vi "Config Seq & Error.vi"(8 "error in (no error)":errorcluster, 11 "Sequences":T1) -> (0 "error out":errorcluster, 3 "Sequences":T1)   [LabVIEW 2014, in "SeqLoop.lvlib"]
uses:
  TypeDefs/Sequence.ctl
  TypeDefs/STEP.ctl
  TypeDefs/LogicParsedExpression.ctl
  Mimico Display/TypeDefs/Mimic Data.ctl
  Mimico Display/TypeDefs/BG Image.ctl
  Mimico Display/TypeDefs/mObject.ctl
  SeqLoop.lvlib
  Mimico Display/Mimico Display.lvlib
panel:
  in  "Save":bool
  in  "Close":bool
  in  "Config AutoZero":bool
  in  "Error&Alarms":bool
  # "Elija la opción que desea configurar"
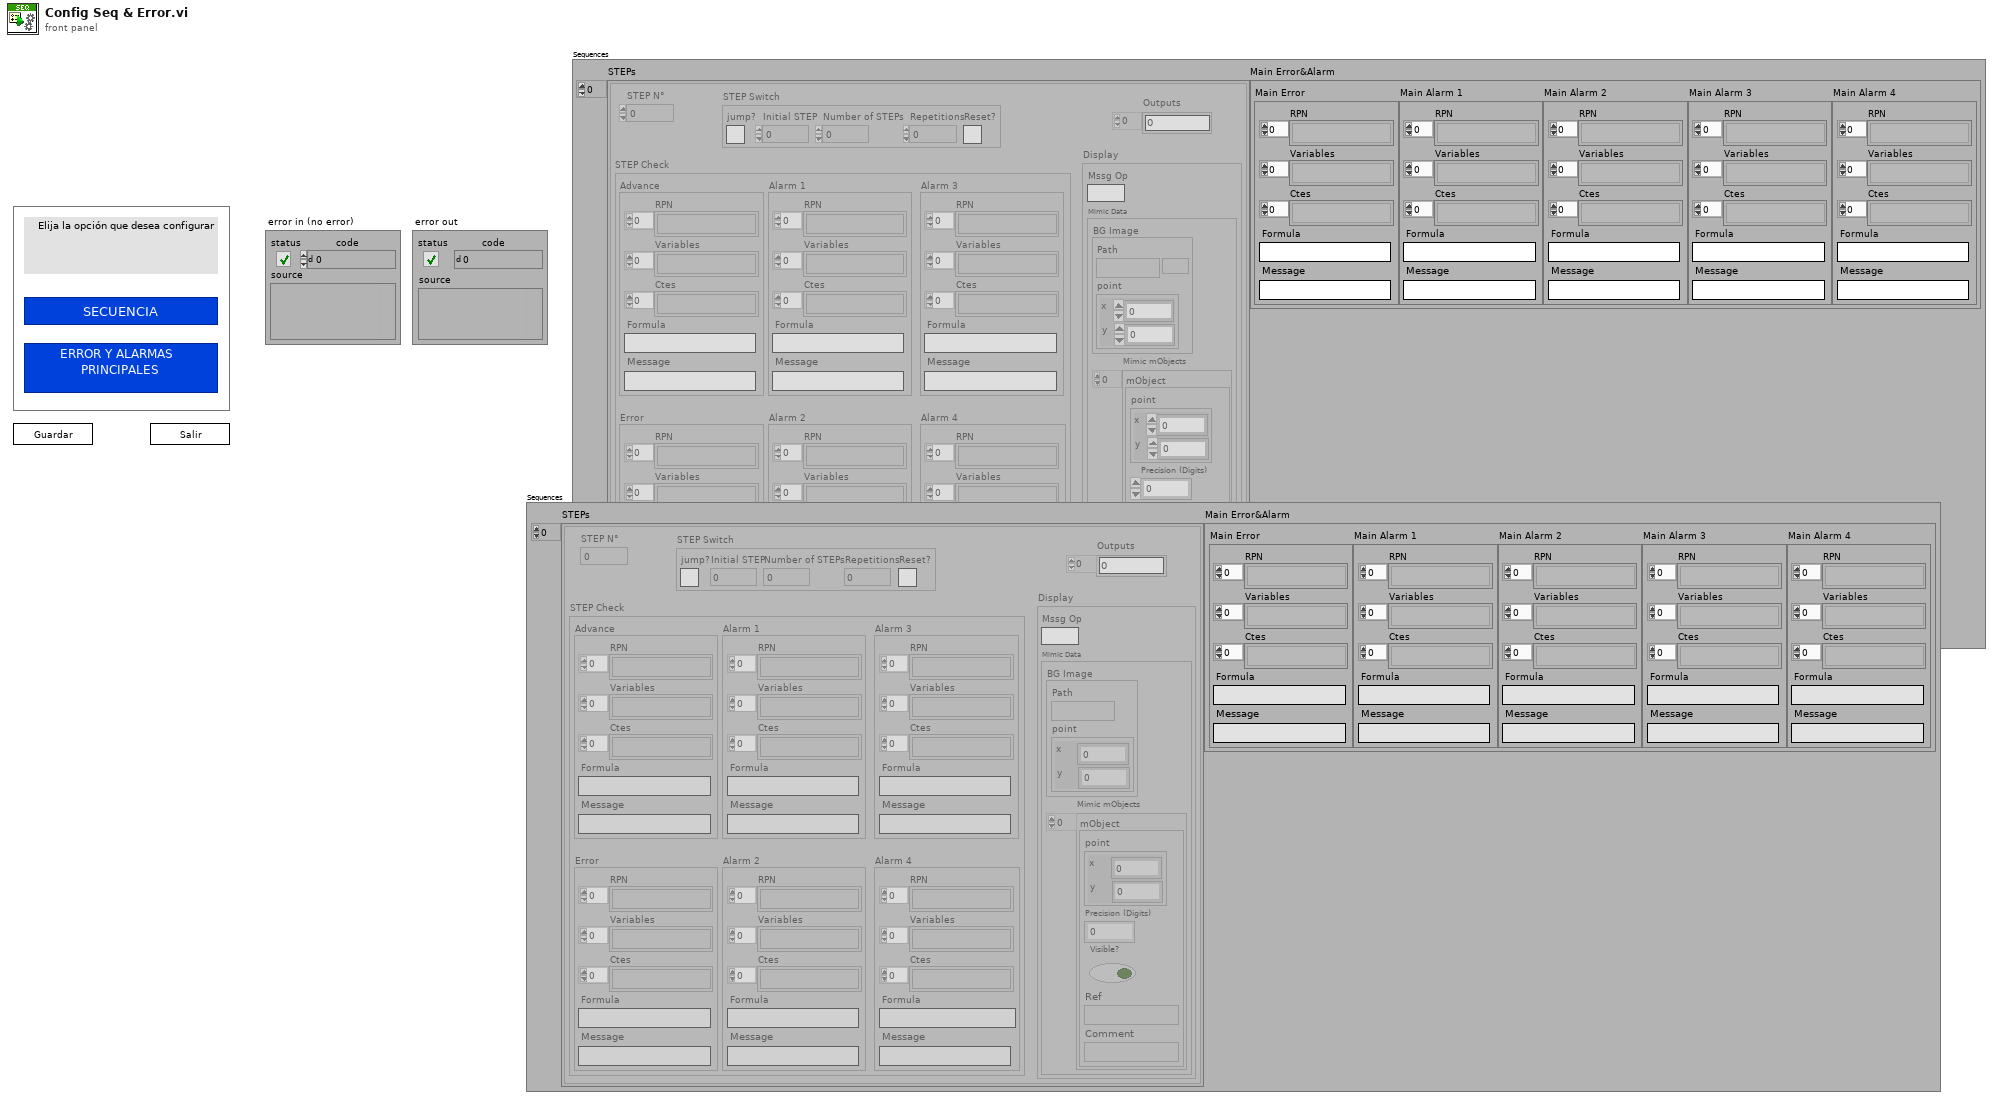
[diagram p1: front panel]
types:
  T1 = typedef "SeqLoop.lvlib/Sequence.ctl" = cluster{"STEPs":T2[], "Main Error&Alarm":cluster{"Main Error":T3, "Main Alarm 1":T3, "Main Alarm 2":T3, "Main Alarm 3":T3, "Main Alarm 4":T3}}
  T2 = typedef "SeqLoop.lvlib/STEP.ctl" = cluster{"STEP N°":u32, "STEP Switch":cluster{"jump?":bool, "Initial STEP":u32, "Number of STEPs":u32, "Repetitions":u32, "Reset?":bool}, "Outputs":i32[], "STEP Check":cluster{"Advance":T3, "Error ":T3, "Alarm 1":T3, "Alarm 2":T3, "Alarm 3":T3, "Alarm 4":T3}, "Display":cluster{"Mssg Op":string, "Mimic Data":T4}}
  T3 = typedef "SeqLoop.lvlib/LogicParsedExpression.ctl" = cluster{"RPN ":string[], "Variables":string[], "Ctes":string[], "Formula":string, "Message":string}
  T4 = typedef "SeqLoop.lvlib/Mimico Display.lvlib/Mimic Data.ctl" = cluster{"BG Image":T5, "Mimic mObjects":T6[]}
  T5 = typedef "SeqLoop.lvlib/Mimico Display.lvlib/BG Image.ctl" = cluster{"Path":path, "point":cluster{"x":i16, "y":i16}}
  T6 = typedef "SeqLoop.lvlib/Mimico Display.lvlib/mObject.ctl" = cluster{"point":cluster{"x":i16, "y":i16}, "Precision (Digits)":i32, "Visible?":bool, "Ref":string, "Comment":string}
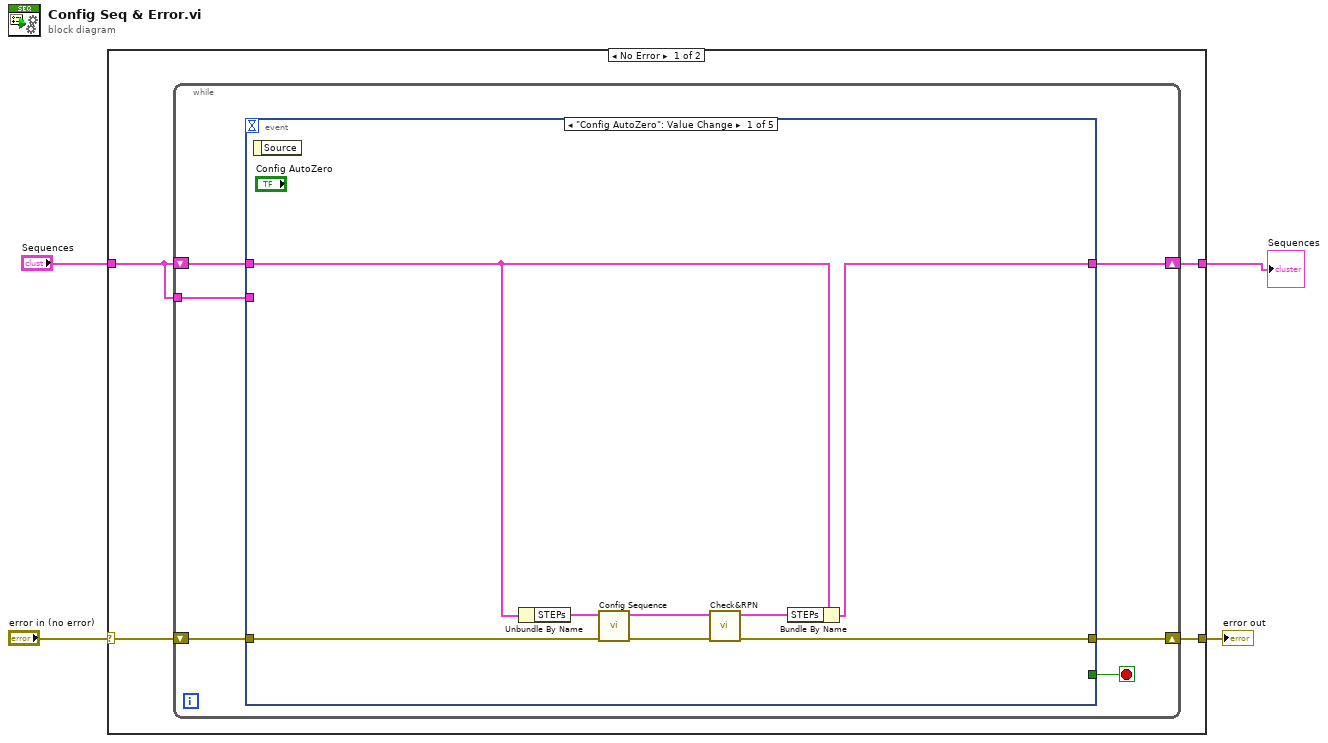
[diagram p0: block diagram]
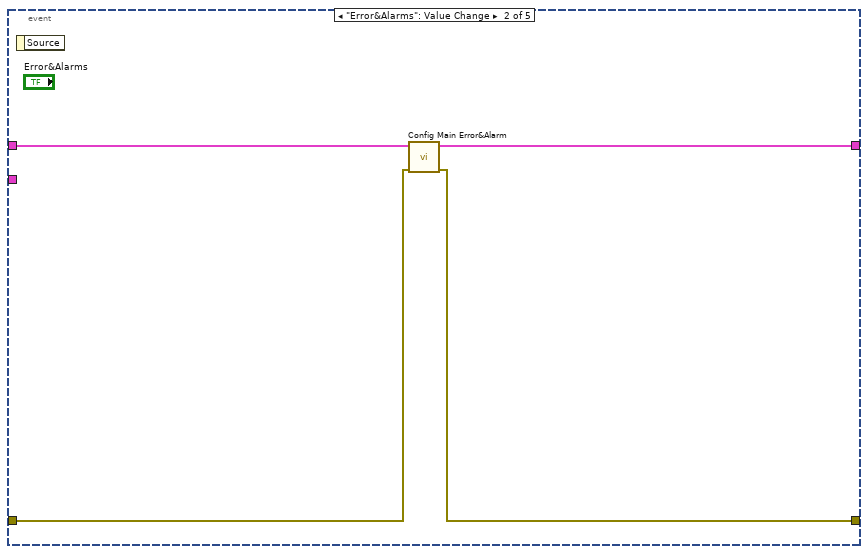
[diagram p2: hidden frame]
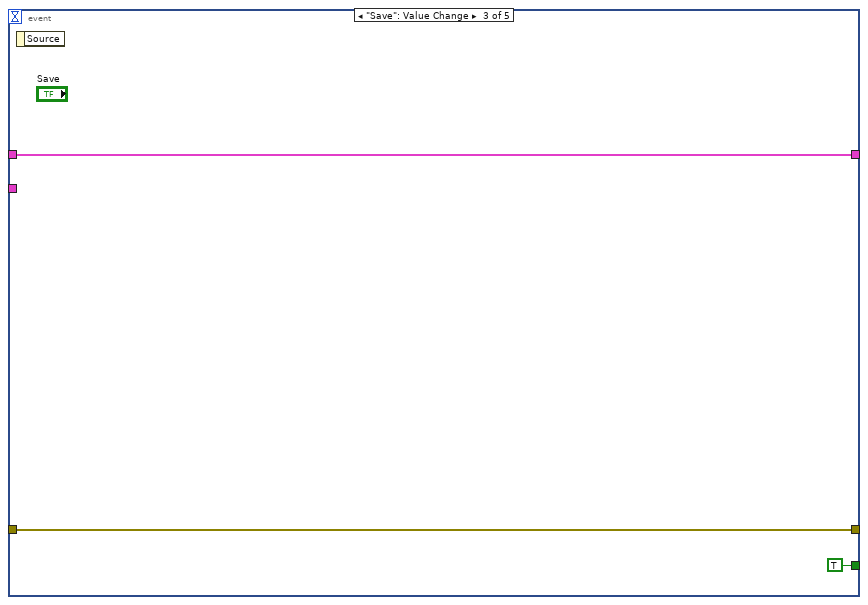
[diagram p3: hidden frame]
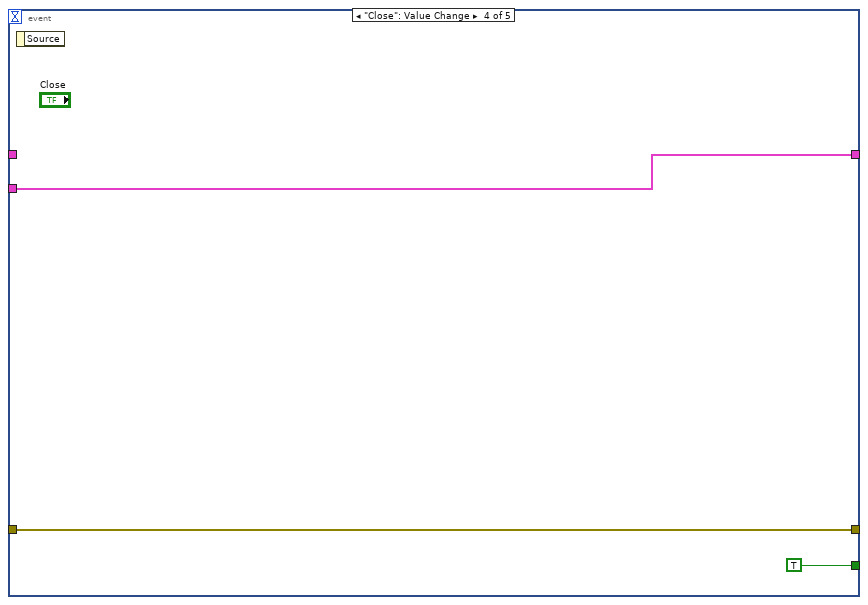
[diagram p4: hidden frame]
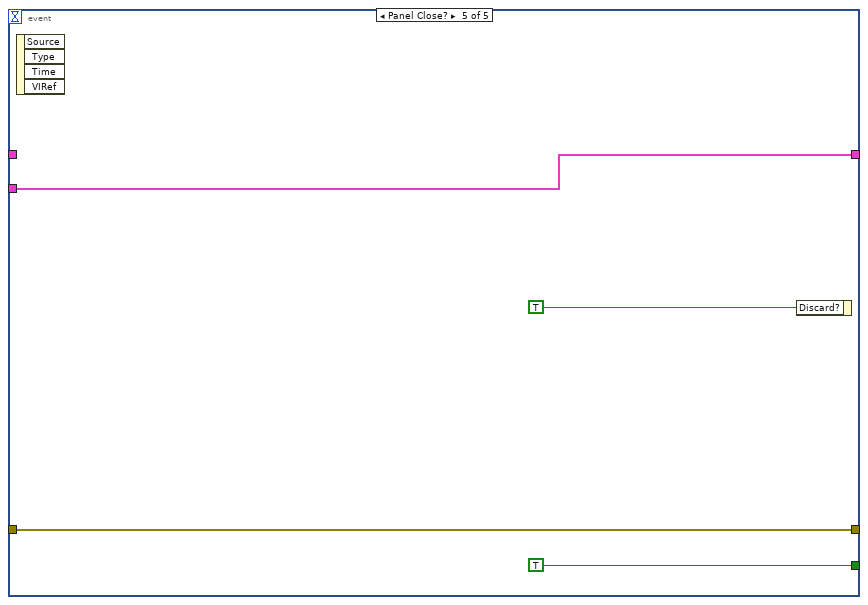
[diagram p5: hidden frame]
diagram:
  n1 = case shown="No Error" "error in (no error)" {
    selector: "error in (no error)" -> [w8 w38]
    tunnel: [w7 w38] -> w3
    tunnel: [w6 w37] -> w2
    tunnel: "Sequences" -> [w5 w37]
    frame No Error {
      n2 = while {
        shift-right: [w13] -> w7
        shift-left: w8 -> [w14]
        shift-right: [w12] -> w6
        shift-left: w5 -> [w11]
        tunnel: w5 -> [w9]
        stop <- w10 stop-if-true
        n3 = event shown="[0] \"Config AutoZero\": Value Change" {
          selector: _ -> [_ _ _ _ _]
          dyn-events: _ -> [_ _ _ _ _]
          timeout: _ -> [_ _ _ _ _]
          tunnel: w14 -> [w21 w23 w27 w32 w34]
          tunnel: [w20 w24 w27 w32 w34] -> w13
          tunnel: [w19 w25 w29 w30 w33] -> w12
          tunnel: w11 -> [w15 w26 w29 _ _]
          tunnel: [_ _ TRUE TRUE TRUE] -> w10
          tunnel: w9 -> [_ _ _ w30 w33]
          event "Config AutoZero": Value Change {
            n4 = event-data() -> ()  [unwired: 1 in, 1 out]
            n5 = Unbundle By Name(w15) -> ("STEPs"=w18:T2[])
            n6 = call "Config Sequence.vi"("error in (no error)"=w21, "STEPs"=w18) -> ("error out"=w22:errorcluster, "STEPs Out"=w17:T2[])  [unwired: 8 in]
            n7 = call "Check&RPN.vi"("error in (no error)"=w22, "Array STEP"=w17) -> ("error out"=w20:errorcluster, "Array STEP Out"=w16:T2[])  [unwired: 8 in]
            n8 = Bundle By Name(cluster=w15, "STEPs"=w16) -> (w19:T1)
          }
          event "Error&Alarms": Value Change {
            n9 = event-data() -> ()  [unwired: 1 in, 1 out]
            n10 = call "Config Main Error&Alarm.vi"("error in (no error)"=w23, "Sequence"=w26) -> ("error out"=w24:errorcluster, "Sequence out"=w25:T1)  [unwired: 8 in]
          }
          event "Save": Value Change {
            n11 = event-data() -> ()  [unwired: 1 in, 1 out]
          }
          event "Close": Value Change {
            n12 = event-data() -> ()  [unwired: 1 in, 1 out]
          }
          event Panel Close? {
            n13 = event-data() -> ()  [unwired: 1 in, 4 out]
            n14 = event-data("Discard?"=TRUE) -> ()  [unwired: 1 in, 1 out]
          }
        }
      }
    }
    frame Error {
    }
  }
  "error out" <- w3
  "Sequences" <- w2
